vi "Create.vi"(8 "error in (no error)":errorcluster, 10 "components directory":path, 11 "Component Loader type":refnum<class "Component Loader.lvclass">) -> (0 "error out":errorcluster, 3 "Component Loader out":refnum<class "Component Loader.lvclass">)   [LabVIEW 2019, in "DSF Core.lvlib" / "Component Loader.lvclass"]
uses:
  Component Loader.lvclass
  Component Loader.lvclass/Component Loader.ctl
  Component Directory Not Found.vi
  New Component Loader Error.vi
  <vilib>/NI/Memory Manager/VIs/Write String to Source.vi
  <vilib>/NI/Memory Manager/VIs/New Error Cluster.vi
  <vilib>/NI/Memory Manager/VIs/New Error Cluster (512B).vi
  Component Loader Error Info.vi
  <vilib>/NI/Memory Manager/VIs/Set Error Code.vi
  <vilib>/NI/Memory Manager/VIs/Set Error Status.vi
  <vilib>/NI/Memory Manager/VIs/Set Error Source.vi
  VIs/Constants/Constants.vi
  VIs/Constants/Engine Library Name.vi
  Base Error Offset.vi
  VIs/Constants/Base Error Code.vi
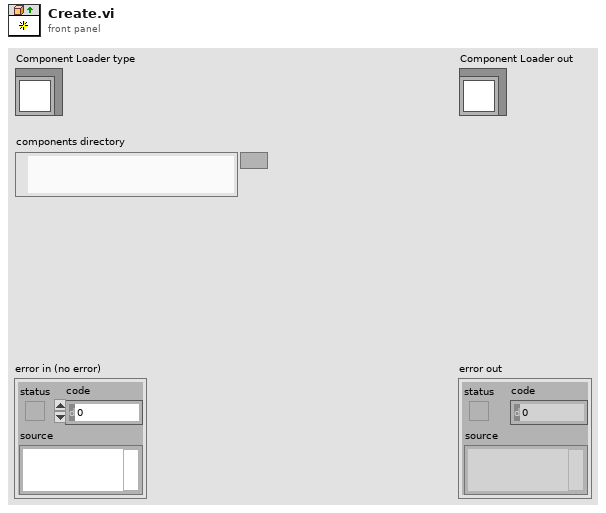
[diagram p1: front panel]
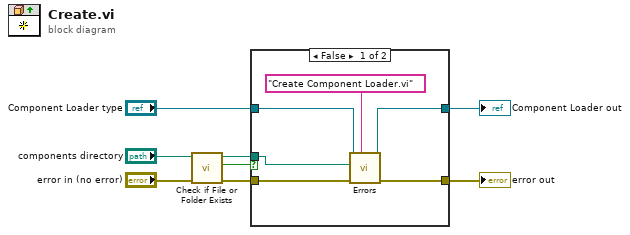
[diagram p0: block diagram]
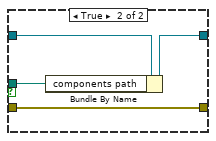
[diagram p2: hidden frame]
diagram:
  n1 = call <vilib>:"Check if File or Folder Exists.vi"("error in (no error)"="error in (no error)", "path"="components directory") -> ("error out"=w5:errorcluster, "file or folder exists?"=w3:bool, "dup path"=w6:path)  [unwired: 7 in]
  n2 = case shown="False" w3 {
    tunnel: "Component Loader type" -> [w12 w18]
    tunnel: [w11 w17] -> w7
    tunnel: w6 -> [w10 w16]
    tunnel: w5 -> [w14 w15]
    tunnel: [w13 w15] -> w4
    frame False {
      n3 = call-poly "Errors.vi"("error source vi name"="Create Component Loader.vi", "error in (no error)"=w14, "configured path"=w10, "Component Loader in"=w12) -> ("error out"=w13:errorcluster, "Component Loader out"=w11:refnum<class "Component Loader.lvclass">)  [unwired: 6 in]
    }
    frame True {
      n4 = Bundle By Name(cluster=w18, "components path"=w16) -> (w17:refnum<class "Component Loader.lvclass">)
    }
  }
  "error out" <- w4
  "Component Loader out" <- w7
